vi "ArrayExercise.vi"() -> ()   [LabVIEW 2025]
panel:
  out "Subset Array":dbl[](array[numeric])
  in  "# of Elements":i32
  in  "Start Subset":i32
  in  "Scaling Factor":dbl
  out "Final Array":dbl[](array[numeric])
  out "Random Array":dbl[](array[numeric])
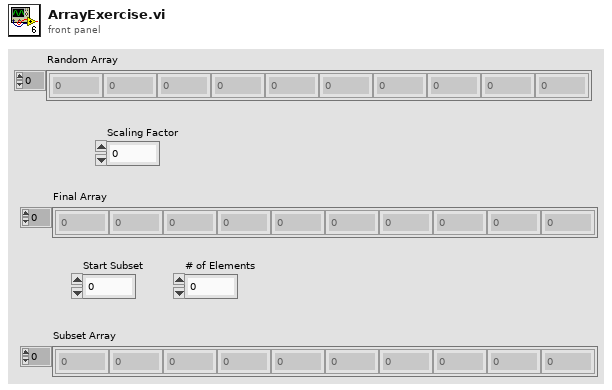
[diagram p1: front panel]
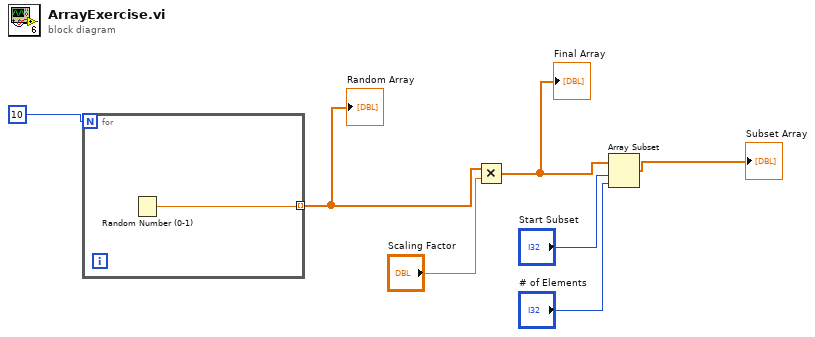
[diagram p0: block diagram]
diagram:
  n1 = for {
    N: 10 -> [_]
    tunnel: [w8] -> w6 mode=indexing
    n2 = Random Number (0-1)() -> (number: 0 to 1=w8:dbl)
  }
  "Random Array" <- w6
  n3 = Multiply(x=w6, y="Scaling Factor") -> (x*y=w4:dbl[])
  "Final Array" <- w4
  n4 = Array Subset(array=w4, index="Start Subset", length="# of Elements") -> (→"Subset Array":dbl[])
